vi "Write meta data.vi"(8 "error in":errorcluster, 9 "timeout ms (25000)":i32=25000, 10 "Meta data":string[](array[string]), 11 "connection ID":refnum<k5>) -> (0 "error out":errorcluster, 3 "Connection Info":T1)   [LabVIEW 2021]
uses:
  Connection Info.ctl
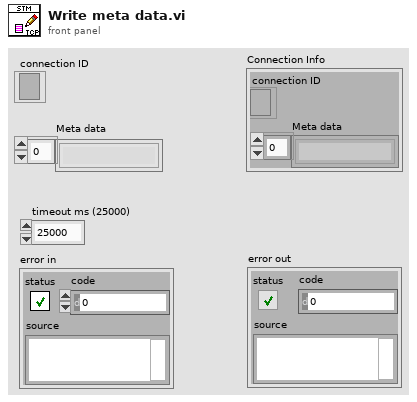
[diagram p1: front panel]
types:
  T1 = typedef "Connection Info.ctl" = cluster{"connection ID":refnum<k5>, "Meta data":string[]}
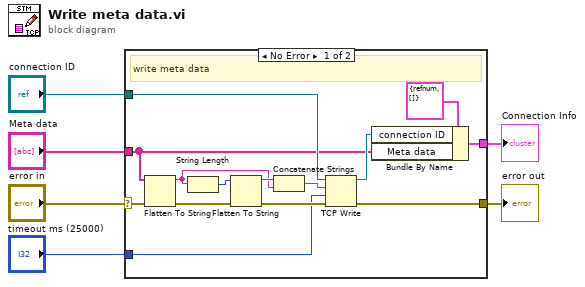
[diagram p0: block diagram]
diagram:
  n1 = case shown="No Error" "error in" {
    selector: "error in" -> [w15 w21]
    tunnel: "connection ID" -> [w17 _]
    tunnel: "Meta data" -> [w10 _]
    tunnel: "timeout ms (25000)" -> [w12 _]
    tunnel: [w9 _] -> w2
    tunnel: [w8 w21] -> w1
    frame No Error {
      # "write meta data"
      n2 = Flatten To String(anything=w10, error in (no error)=w15) -> (data string=w18:string, error out=w14:errorcluster)  [unwired: 2 in, 1 out]
      n3 = String Length(string=w18) -> (length=w20:i32)
      n4 = Flatten To String(anything=w20, error in (no error)=w14) -> (data string=w19:string, error out=w13:errorcluster)  [unwired: 2 in, 1 out]
      n5 = Concatenate Strings(w19, w18) -> (w16:string)
      n6 = TCP Write(connection ID=w17, data in=w16, error in (no error)=w13, 9:w12) -> (connection ID out=w11:refnum<k5>, error out=w8:errorcluster)  [unwired: 1 out]
      n7 = Bundle By Name(cluster=T1 {"connection ID"=refnum, "Meta data"=[]} ("Connection Info"), "connection ID"=w11, "Meta data"=w10) -> (w9:T1)
    }
    frame Error {
    }
  }
  "Connection Info" <- w2
  "error out" <- w1
